vi "testFringeViewer.vi"() -> ()   [LabVIEW 2009, in "run.lvlib"]
uses:
  run.lvlib
panel:
  out "XY Graph":cluster{dbl[], dbl[]}(graph)
  in  "stop":bool=TRUE
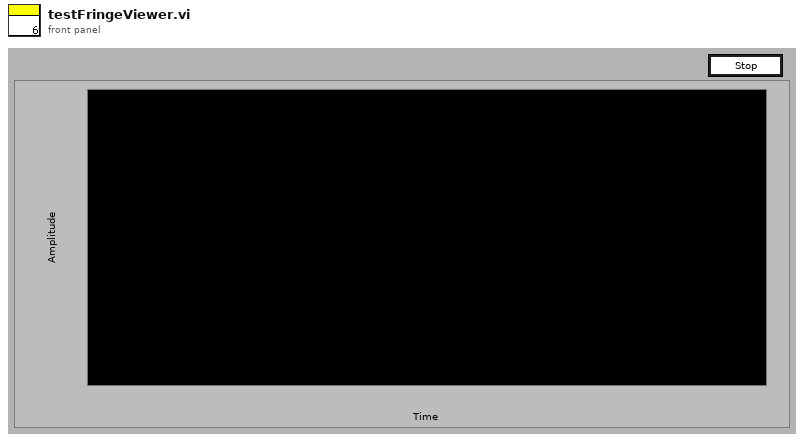
[diagram p1: front panel]
types:
  T1 = cluster{"Name":string, "Results":dbl[], "AnalysisType":string}
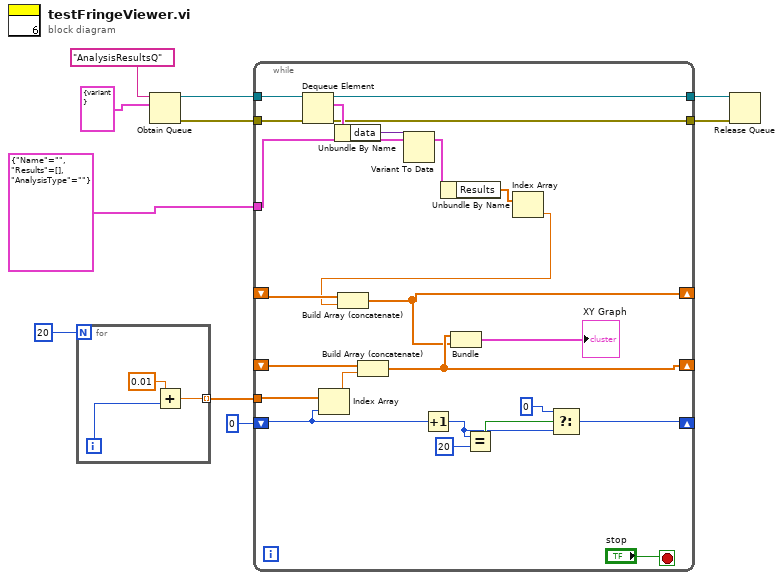
[diagram p0: block diagram]
diagram:
  n1 = for {
    N: 20 -> [_]
    tunnel: [w11] -> w4 mode=indexing
    i -> [w12]
    n2 = Add(x=0.01, y=w12) -> (x+y=w11:dbl)
  }
  n3 = Obtain Queue(name (unnamed)="AnalysisResultsQ", element data type=cluster{"data":variant} {"data"=variant} ("dataQ")) -> (queue out=w9:refnum<queue>, error out=w8:errorcluster)  [unwired: 3 in, 1 out]
  n4 = while {
    tunnel: w9 -> [w23]
    tunnel: w8 -> [w22]
    tunnel: T1 {"Name"="", "Results"=[], "AnalysisType"=""} ("output cluster") -> [w18]
    tunnel: w4 -> [w35]
    shift-right: [w32] -> _
    shift-left: _ -> [w34]
    shift-right: [w31] -> _
    shift-left: _ -> [w30]
    shift-right: [w28] -> _
    shift-left: 0 -> [w29]
    tunnel: [w15] -> w2
    tunnel: [w14] -> w1
    stop <- "stop" stop-if-true
    n5 = Dequeue Element(queue=w23, error in (no error)=w22) -> (queue out=w15:refnum<queue>, element=w21:cluster{"data":variant}, error out=w14:errorcluster)  [unwired: 1 in, 1 out]
    n6 = Index Array(array=w35, index=w29) -> (element=w33:dbl)
    n7 = Unbundle By Name(w21) -> ("data"=w20:variant)
    n8 = Build Array (concatenate)(w34, w33) -> (w32:dbl[])
    n9 = Variant To Data(Variant=w20, type=w18) -> (data=w19:T1)  [unwired: 1 in, 1 out]
    n10 = Increment(x=w29) -> (x+1=w26:i32)
    n11 = Unbundle By Name(w19) -> ("Results"=w17:dbl[])
    n12 = Equal?(x=w26, y=20) -> (x = y?=w27:bool)
    n13 = Index Array(array=w17) -> (element=w16:dbl)  [unwired: 1 in]
    n14 = Build Array (concatenate)(w30, w16) -> (w31:dbl[])
    n15 = Bundle(w32, w31) -> (→"XY Graph":cluster{dbl[], dbl[]})  [unwired: 1 in]
    n16 = Select(t=0, s=w27, f=w26) -> (s? t:f=w28:i32)
  }
  n17 = Release Queue(queue=w2, error in (no error)=w1) -> ()  [unwired: 1 in, 3 out]
